vi "Add Acknowledge Bit.vi"(8 "error in (no error)":errorcluster, 10 "Action":T1, 11 "I2C waveform info":T2) -> (0 "error out":errorcluster, 3 "I2C waveform info out":T2)   [LabVIEW 2009, in "IDW.lvlib"]
doc: "Adds an acknowledge (ACK) bit to the I2C waveform.\n\nFor a <b>Listen</b> action, the SDA line is released and a single sample in the center of the clock pulse is compared against the expected value. For a <b>Send</b> action, the value is written to the SDA line according to the timing parameters specified by the <b>Init</b> VI.\n\nTiming parameters that affect this waveform segment's length are: <b>tSU;DAT</b>, <b>tHIGH</b>, and <b>tHD;DAT</b>."
uses:
  IDW.lvlib
  _Typedefs/Waveform info.ctl
  _Typedefs/Timing - ticks.ctl
  _Typedefs/Default transition action.ctl
  _Typedefs/Bit type.ctl
  _Typedefs/ACK action.ctl
  _Typedefs/Transition action.ctl
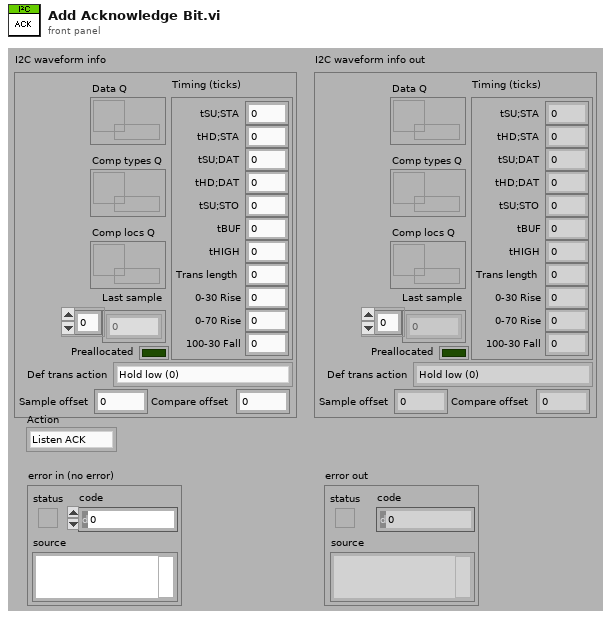
[diagram p1: front panel]
types:
  T1 = typedef "IDW.lvlib/ACK action.ctl" = enum16{"Listen ACK", "Listen NACK", "Send ACK", "Send NACK"}
  T2 = typedef "IDW.lvlib/Waveform info.ctl" = cluster{"Last sample":u8[], "Sample offset":u64, "Compare offset":u64, "Timing (ticks)":T3, "Preallocated":bool, "Def trans action":T4, "Data Q":refnum<queue>, "Comp types Q":refnum<queue>, "Comp locs Q":refnum<queue>}
  T3 = typedef "IDW.lvlib/Timing - ticks.ctl" = cluster{"tSU;STA":i32, "tHD;STA":i32, "tSU;DAT":i32, "tHD;DAT":i32, "tSU;STO":i32, "tBUF":i32, "tHIGH":i32, "Trans length":i32, "0-30 Rise":i32, "0-70 Rise":i32, "100-30 Fall":i32}
  T4 = typedef "IDW.lvlib/Default transition action.ctl" = enum16{"Hold low (0)", "Release (Z)", "Set up next value", "Hold previous value", "Preserve tHD;DAT and tSU;DAT"}
  T5 = typedef "IDW.lvlib/Transition action.ctl" = enum16{"Hold low (0)", "Release (Z)", "Set up next value", "Hold previous value", "Preserve tHD;DAT and tSU;DAT", "<Use session default>"}
  T6 = typedef "IDW.lvlib/Bit type.ctl" = enum16{"ACK", "Data"}
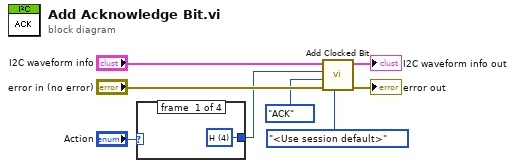
[diagram p0: block diagram]
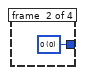
[diagram p2: hidden frame]
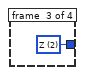
[diagram p3: hidden frame]
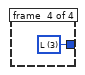
[diagram p4: hidden frame]
diagram:
  n1 = case shown="\"Listen ACK\", Default" "Action" {
    tunnel: [w9 w10 w11 w12] -> w4
    frame #0 {
      w9 = u8 4 items=["0", "1", "Z", "L", "H", "X", "T", "V"] ("Bit")
    }
    frame #1 {
      w10 = u8 0 items=["0", "1", "Z", "L", "H", "X", "T", "V"] ("Bit")
    }
    frame #2 {
      w11 = u8 2 items=["0", "1", "Z", "L", "H", "X", "T", "V"] ("Bit")
    }
    frame #3 {
      w12 = u8 3 items=["0", "1", "Z", "L", "H", "X", "T", "V"] ("Bit")
    }
  }
  n2 = call "Add Clocked Bit.vi"("Transition action"=Transition_action."<Use session default>", "error in (no error)"="error in (no error)", "Bit type"=Bit_type."ACK", "Bit value"=w4, "I2C waveform info"="I2C waveform info") -> ("error out"=→"error out":errorcluster, "I2C waveform info out"=→"I2C waveform info out":T2)  [unwired: 5 out]
